vi "Set Kernel Arguments uint.vi"(7 "Local Data?":bool, 8 "Error In":errorcluster, 9 "Kernel Handle":T1, 10 "Argument Number":i32, 11 "uint Constant":u32[](array[numeric])) -> (0 "Error Out":errorcluster, 1 "Kernel Handle out":T1, 2 "Auto Inc Arugment Number":i32)   [LabVIEW 2012, in "OpenCLV x64.lvlib"]
doc: "Sets an argument of a kernel to a i32 (uint) constant. Can also be used to set vector constants.\n\nFor example, if a kernel requires uint Constant, convert the constant in Labview into a 1D array and pass the constant into this VI. If a kernel requires uint4 Constant, simply wire the 1D array of uint constants into this VI.\n\nThis VI may also be used to allocate local memory for a kernel for use with Work Groups. If a kernel requires __local uint *LocalMem that is 512 uint values, allocate a 1D array of uint numbers in Labview and pass them into this VI and also set <b>Local Data?</b> to true. <b>No data is transferred to the device with this VI in this configuration.</b>"
uses:
  OpenCLV x64.lvlib
  Controls/Kernel Handle.ctl
  Error Checking/Add Error Functional Global.vi
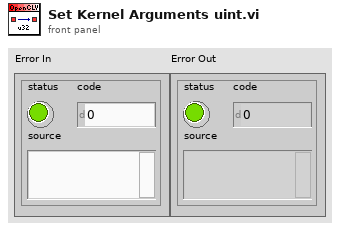
[diagram p1: front panel]
types:
  T1 = typedef "OpenCLV x64.lvlib/Kernel Handle.ctl" = u64
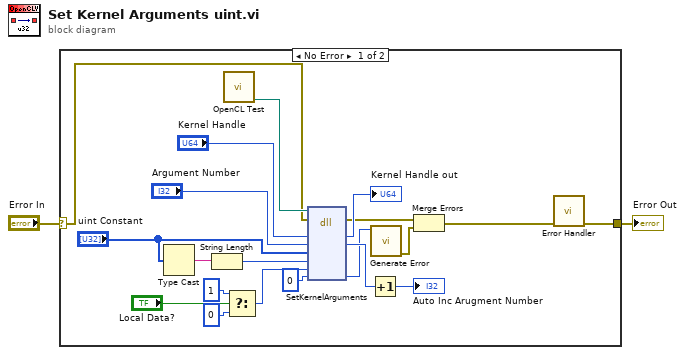
[diagram p0: block diagram]
diagram:
  n1 = case shown="No Error" "Error In" {
    selector: "Error In" -> [w3 w23]
    tunnel: [w7 w23] -> w1
    frame No Error {
      n2 = Type Cast(x="uint Constant") -> (*(type *) &x=w18:string)  [unwired: 1 in]
      n3 = String Length(string=w18) -> (length=w16:i32)
      n4 = call "OpenCL Test.vi"() -> ("DLL To Use"=w8:path)  [unwired: 11 in]
      n5 = Select(t=1, s="Local Data?", f=0 ("t")) -> (s? t:f=w9:i32)
      n6 = dll-call lib="C:/Users/bme-amcelroy-la/Desktop/OpenCLV/trunk/OpenCLV_x64_1.0/OpenCLV_x64.dll" fn="SetKernelArguments"(path in=w8, error in=w3, "Kernel Handle"="Kernel Handle", "Argument Number"="Argument Number", "Data"="uint Constant", "Size of Data Pointer in bytes"=w16, "Local"=w9, "Error"=0) -> (error out=w4:errorcluster, "Kernel Handle"=→"Kernel Handle out":u64, "Argument Number"=w14:i32, "Error"=w13:i32)  [unwired: 5 in, 1 out]
      n7 = Increment(x=w14) -> (x+1=→"Auto Inc Arugment Number":i32)
      n8 = call "Generate Error.vi"("Error"=w13) -> ("error out"=w6:errorcluster)  [unwired: 10 in]
      n9 = Merge Errors(w4, w6) -> (w5:errorcluster)
      n10 = call-poly "Error Handler.vi"("Error In"=w5) -> ("Error Out"=w7:errorcluster)  [unwired: 10 in]
    }
    frame Error {
    }
  }
  "Error Out" <- w1
